vi "Ohmmeter.vi"() -> ()   [LabVIEW 2020]
uses:
  CircuitParameters.ctl
  <vilib>/MakerHub/LINX/Public/Peripherals/Analog/Analog Read 1 Chan.vi
  <vilib>/MakerHub/LINX/Public/Peripherals/Analog/Analog Read N Chans.vi
  <vilib>/MakerHub/LINX/Private/Local IO/LinxAnalogRead.vi
  <vilib>/MakerHub/LINX/Public/Utilities/Check Channel.vi
  <vilib>/MakerHub/LINX/Public/Utilities/Open Serial.vi
  <vilib>/MakerHub/LINX/Private/Utilties/Generate Error.vi
  <vilib>/MakerHub/LINX/LMH-LINX.lvlib
panel:
  out "Measurements History":dbl[](graph)
  out "Device Name":string
  in  "Circuit Parameters 2":T1
  in  "Measurements by Seconds":dbl
  in  "Analog Pin":u8
  in  "Serial Port":refnum<visa-resource-name>="N/A"
  in  "Pause Measurements":bool
  in  "Save Data As CSV":bool
  in  "Stop Application":bool
  in  "Record Measurements":bool
  # "Serial Communication \nParameters"
  # "Measurements"
  # "Circuit Parameters"
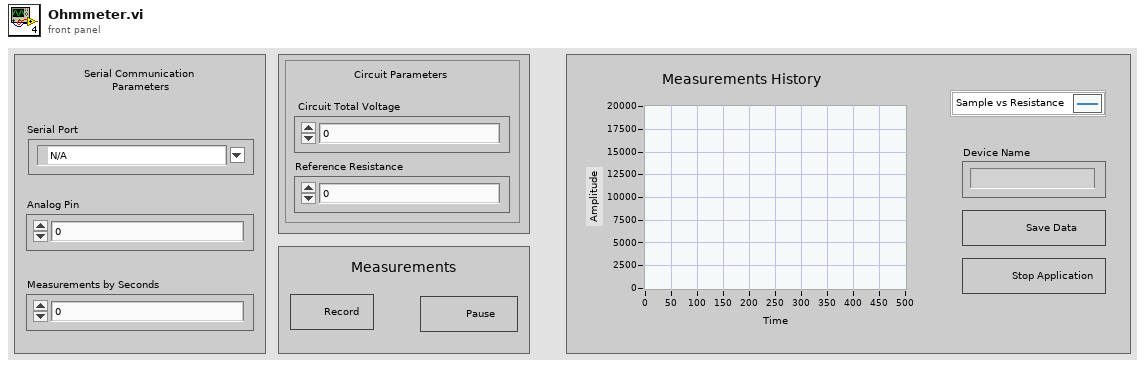
[diagram p1: front panel]
types:
  T1 = typedef "CircuitParameters.ctl" = cluster{"Reference Resistance":dbl, " Circuit Total Voltage":dbl}
  T2 = typedef "LMH-LINX.lvlib/LINX Ref.ctl" = cluster{"IO":T3, "Interface":T4, "LINX Device Config":T5}
  T3 = typedef "LMH-LINX.lvlib/Platform.ctl" = enum16{"Remote", "Local"}
  T4 = typedef "LMH-LINX.lvlib/Interface.ctl" = enum16{"Serial", "TCP"}
  T5 = typedef "LMH-LINX.lvlib/Device.lvlib/LINX Device Config.ctl" = cluster{"Interface":T4, "COM Port":refnum<visa-resource-name>, "TCP Configuration":T6, "Device Family":u8, "Device ID":u8, "Device Name":string, "TCP Ref":refnum<k5>, "Channels":T7}
  T6 = typedef "LMH-LINX.lvlib/Device.lvlib/TCP Config.ctl" = cluster{"IP Address":string, "Port":u16}
  T7 = typedef "LMH-LINX.lvlib/Channels.ctl" = cluster{"DI":u8[], "DO":u8[], "AI":u8[], "AO":u8[], "PWM":u8[], "QE":u8[], "UART":u8[], "I2C 2":u8[], "SPI":u8[], "CAN":u8[], "Servo":u8[], "AI Ref (V)":dbl, "AI Resolution (Bits)":u8, "AO Ref (V)":dbl, "AO Resolution (Bits)":u8}
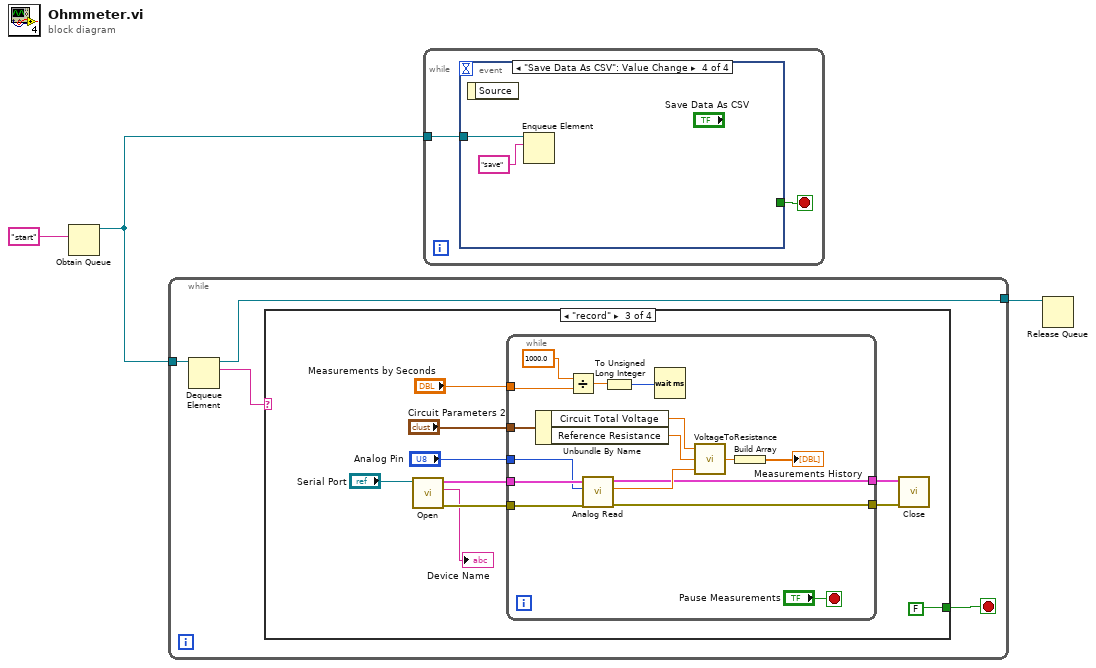
[diagram p0: block diagram]
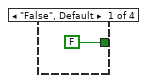
[diagram p2: hidden frame]
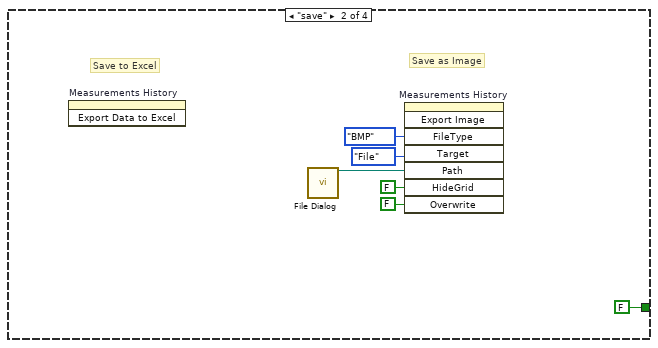
[diagram p3: hidden frame]
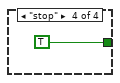
[diagram p4: hidden frame]
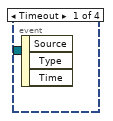
[diagram p5: hidden frame]
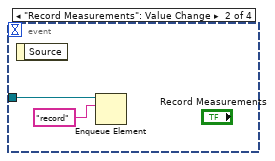
[diagram p6: hidden frame]
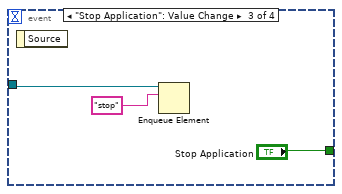
[diagram p7: hidden frame]
diagram:
  n1 = Obtain Queue(element data type="start") -> (queue out=w2:refnum<queue>)  [unwired: 4 in, 2 out]
  n2 = while {
    tunnel: w2 -> [w7]
    tunnel: [w4] -> w1
    stop <- w5 stop-if-true
    n3 = Dequeue Element(queue=w7) -> (queue out=w4:refnum<queue>, element=w6:string)  [unwired: 2 in, 2 out]
    n4 = case shown="\"record\"" w6 {
      tunnel: [FALSE FALSE FALSE TRUE] -> w5
      frame "False", Default {
      }
      frame "save" {
        # "Save as Image"
        # "Save to Excel"
        n5 = invoke on="Measurements History" class="WFChart (strict)" method="Export Data to Excel"() -> ()  [unwired: 3 in, 3 out]
        n6 = call "File Dialog"() -> ("selected path"=w11:path)  [unwired: 12 in, 3 out]
        n7 = invoke on="Measurements History" class="WFChart (strict)" method="Export Image"("FileType"=enum32{"BMP", "EPS", "EMF", "PICT"}."BMP" ("File Type"), "Target"=enum32{"File", "Clipboard"}."File", "Path"=w11, "HideGrid"=FALSE ("Hide Grid"), "Overwrite"=FALSE ("Always Overwrite")) -> ()  [unwired: 3 in, 8 out]
      }
      frame "record" {
        n8 = call-poly <vilib>:"Open.vi"("Serial Port"="Serial Port") -> ("Error Out"=w21:errorcluster, "Device Name"=→"Device Name":string, "LINX Resource"=w23:T2)  [unwired: 8 in]
        n9 = while {
          tunnel: w23 -> [w40]
          tunnel: "Analog Pin" -> [w39]
          tunnel: w21 -> [w38]
          tunnel: "Circuit Parameters 2" -> [w37]
          tunnel: "Measurements by Seconds" -> [w32]
          tunnel: [w28] -> w18
          tunnel: [w27] -> w17
          stop <- "Pause Measurements" stop-if-true
          n10 = Unbundle By Name(w37) -> ("Circuit Total Voltage"=w36:dbl, "Reference Resistance"=w35:dbl)
          n11 = Divide(x=1000.0, y=w32) -> (x/y=w31:dbl)
          n12 = call-poly <vilib>:"Analog Read.vi"("Error In"=w38, "Analog Channel"=w39, "LINX Resource"=w40) -> ("Error Out"=w27:errorcluster, "Voltage"=w34:dbl, "LINX Resource"=w28:T2)  [unwired: 5 in, 1 out]
          n13 = To Unsigned Long Integer(number=w31) -> (unsigned 32bit integer=w30:u32)
          n14 = Wait (ms)(milliseconds to wait=w30) -> ()  [unwired: 1 out]
          n15 = call "VoltageToResistance.vi"("Voltage Measured"=w34, "Reference Resistance (ohms)"=w35, "Circuit Total Voltage (V)"=w36) -> ("Resistance Measured (ohms)"=w29:dbl)
          n16 = Build Array(w29) -> (→"Measurements History":dbl[])
        }
        n17 = call <vilib>:"Close.vi"("Error In"=w17, "LINX Resource"=w18) -> ()  [unwired: 9 in, 1 out]
      }
      frame "stop" {
      }
    }
  }
  n18 = while {
    tunnel: w2 -> [w43]
    stop <- w42 stop-if-true
    n19 = event shown="[3] \"Save Data As CSV\": Value Change" {
      selector: _ -> [_ _ _ _]
      dyn-events: _ -> [_ _ _ _]
      timeout: _ -> [_ _ _ _]
      tunnel: w43 -> [_ w45 w47 w49]
      tunnel: [_ _ "Stop Application" _] -> w42
      event Timeout {
        n20 = event-data() -> ()  [unwired: 1 in, 3 out]
      }
      event "Record Measurements": Value Change {
        n21 = event-data() -> ()  [unwired: 1 in, 1 out]
        n22 = Enqueue Element(queue=w45, element="record") -> ()  [unwired: 2 in, 3 out]
      }
      event "Stop Application": Value Change {
        n23 = event-data() -> ()  [unwired: 1 in, 1 out]
        n24 = Enqueue Element(queue=w47, element="stop") -> ()  [unwired: 2 in, 3 out]
      }
      event "Save Data As CSV": Value Change {
        n25 = event-data() -> ()  [unwired: 1 in, 1 out]
        n26 = Enqueue Element(queue=w49, element="save") -> ()  [unwired: 2 in, 3 out]
      }
    }
  }
  n27 = Release Queue(queue=w1) -> ()  [unwired: 2 in, 3 out]
